vi "Save Plot Group Prefs.vi"(8 "error in (no error)":errorcluster, 10 "Plot Group Config":T1, 11 "Pref Group in":refnum<class "Pref Group.lvclass">) -> (0 "error out":errorcluster, 3 "Pref Group out":refnum<class "Pref Group.lvclass">)   [LabVIEW 2020, in "VolatusGUI.lvlib" / "Historian Charting Manager.lvclass"]
uses:
  Historian Charting Manager.lvclass
  lv-userprefs/User Prefs/Pref Group/Pref Group.lvclass
  Plot Group Config.ctl
  X-Axis Type.ctl
  Plot Config.ctl
  Scale.ctl
  Historian Charting Manager.lvclass/Historian Charting Manager.ctl
  lv-vecto/Vecto/Vecto.lvlib
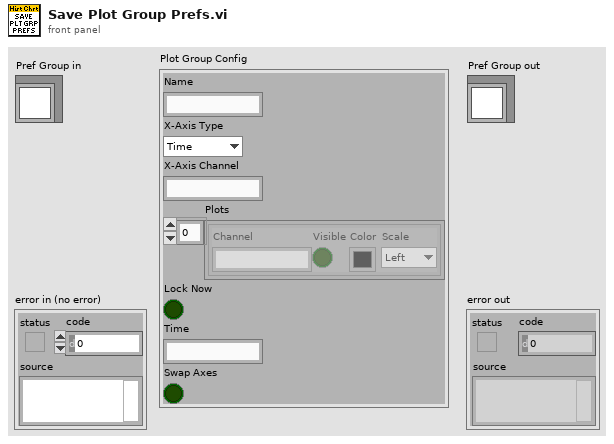
[diagram p1: front panel]
types:
  T1 = typedef "VolatusGUI.lvlib/Historian Charting Manager.lvclass/Plot Group Config.ctl" = cluster{"Name":string, "X-Axis Type":T2, "X-Axis Channel":string, "Plots":T3[], "Lock Now":bool, "Time":string, "Swap Axes":bool}
  T2 = typedef "VolatusGUI.lvlib/Historian Charting Manager.lvclass/X-Axis Type.ctl" = enum16{"Time", "Channel"}
  T3 = typedef "VolatusGUI.lvlib/Historian Charting Manager.lvclass/Plot Config.ctl" = cluster{"Channel":string, "Visible":bool, "Color":u32, "Scale":T4}
  T4 = typedef "VolatusGUI.lvlib/Historian Charting Manager.lvclass/Scale.ctl" = enum16{"Left", "Right"}
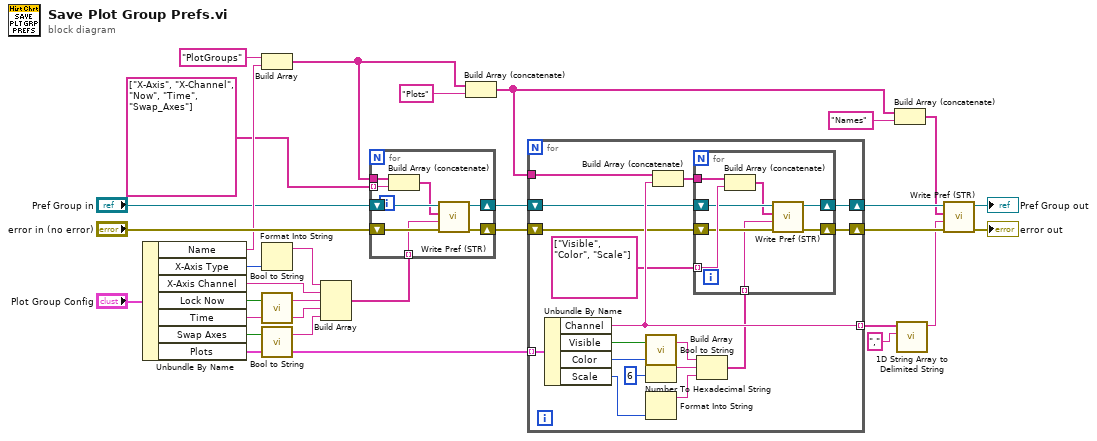
[diagram p0: block diagram]
diagram:
  n1 = Unbundle By Name("Plot Group Config") -> ("Name"=w27:string, "X-Axis Type"=w25:T2, "X-Axis Channel"=w21:string, "Lock Now"=w24:bool, "Time"=w19:string, "Swap Axes"=w23:bool, "Plots"=w15:T3[])
  n2 = Build Array("PlotGroups", w27) -> (w2:string[])
  n3 = Format Into String(w25) -> (resulting string=w22:string)  [unwired: 3 in, 1 out]
  n4 = call "Bool to String.vi"("Bool"=w24) -> ("String"=w20:string)  [unwired: 2 in]
  n5 = call "Bool to String.vi"("Bool"=w23) -> ("String"=w18:string)  [unwired: 2 in]
  n6 = Build Array(w22, w21, w20, w19, w18) -> (w17:string[])
  n7 = for {
    shift-right: [w35] -> w13
    shift-left: "error in (no error)" -> [w38]
    shift-right: [w36] -> w14
    shift-left: "Pref Group in" -> [w37]
    tunnel: w17 -> [w34] mode=indexing
    tunnel: w2 -> [w33]
    tunnel: string[] ["X-Axis", "X-Channel", "Now", "Time", "Swap_Axes"] -> [w32] mode=indexing
    n8 = Build Array (concatenate)(w33, w32) -> (w31:string[])
    n9 = call "Write Pref (STR).vi"("error in (no error)"=w38, "Value"=w34, "Pref Hierarchy"=w31, "Pref Group in"=w37) -> ("error out"=w35:errorcluster, "Pref Group out"=w36:refnum<class "Pref Group.lvclass">)  [unwired: 6 in]
  }
  n10 = Build Array (concatenate)(w2, "Plots") -> (w1:string[])
  n11 = for {
    tunnel: w15 -> [w55] mode=indexing
    shift-right: [w40] -> w8
    shift-left: w14 -> [w45]
    shift-right: [w39] -> w9
    shift-left: w13 -> [w44]
    tunnel: w1 -> [w54]
    tunnel: [w46] -> w11 mode=indexing
    n12 = Unbundle By Name(w55) -> ("Channel"=w46:string, "Visible"=w53:bool, "Color"=w51:u32, "Scale"=w50:T4)
    n13 = call "Bool to String.vi"("Bool"=w53) -> ("String"=w48:string)  [unwired: 2 in]
    n14 = Number To Hexadecimal String(1:i16 6 ("width (-)"), 2:w51) -> (0:w49:string)
    n15 = Format Into String(w50) -> (resulting string=w47:string)  [unwired: 3 in, 1 out]
    n16 = Build Array (concatenate)(w54, w46) -> (w42:string[])
    n17 = Build Array(w48, w49, w47) -> (w41:string[])
    n18 = for {
      shift-right: [w59] -> w40
      shift-left: w45 -> [w60]
      shift-right: [w58] -> w39
      shift-left: w44 -> [w61]
      tunnel: string[] ["Visible", "Color", "Scale"] -> [w62] mode=indexing
      tunnel: w42 -> [w63]
      tunnel: w41 -> [w56] mode=indexing
      n19 = Build Array (concatenate)(w63, w62) -> (w57:string[])
      n20 = call "Write Pref (STR).vi"("error in (no error)"=w61, "Value"=w56, "Pref Hierarchy"=w57, "Pref Group in"=w60) -> ("error out"=w58:errorcluster, "Pref Group out"=w59:refnum<class "Pref Group.lvclass">)  [unwired: 6 in]
    }
  }
  n21 = Build Array (concatenate)(w1, "Names") -> (w4:string[])
  n22 = call <vilib>:"1D String Array to Delimited String.vi"("delimiter"=",", "string array"=w11) -> ("delimited string"=w7:string)  [unwired: 9 in]
  n23 = call "Write Pref (STR).vi"("error in (no error)"=w9, "Value"=w7, "Pref Hierarchy"=w4, "Pref Group in"=w8) -> ("error out"=→"error out":errorcluster, "Pref Group out"=→"Pref Group out":refnum<class "Pref Group.lvclass">)  [unwired: 6 in]
